vi "2 dof inverse.vi"() -> ()   [LabVIEW 2021]
panel:
  out "Motor angles":cluster{"x":dbl, "y":dbl, "x 2":dbl, "y 2":dbl}
  in  "Parameters of 2 DOF":T1={"X"=0.0, "Y"=0.0, "l1"=230.59, "l2"=112.96, "phi (rad)"=112.96} caption="Parameters of Delta Robot"
  # "Definitions about the Inputs of Forward Kinematics :"
  # "Theta Motor 1 , Theta Motor 2 represents the angles of two smart motors of 2 DOF."
  # "l1 and l2 respresents links length."
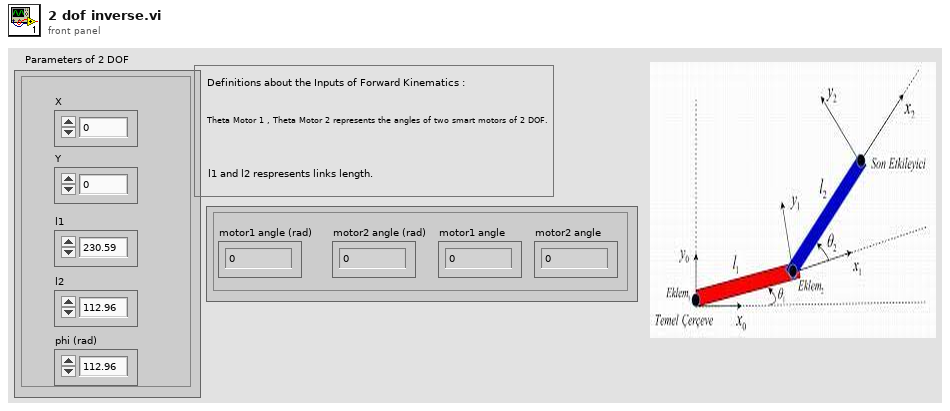
[diagram p1: front panel]
types:
  T1 = cluster{"X":dbl, "Y":dbl, "l1":dbl, "l2":dbl, "phi (rad)":dbl}
  T2 = cluster{"theta1":dbl, "theta2":dbl, "theta1_dg":dbl, "theta2_dg":dbl}
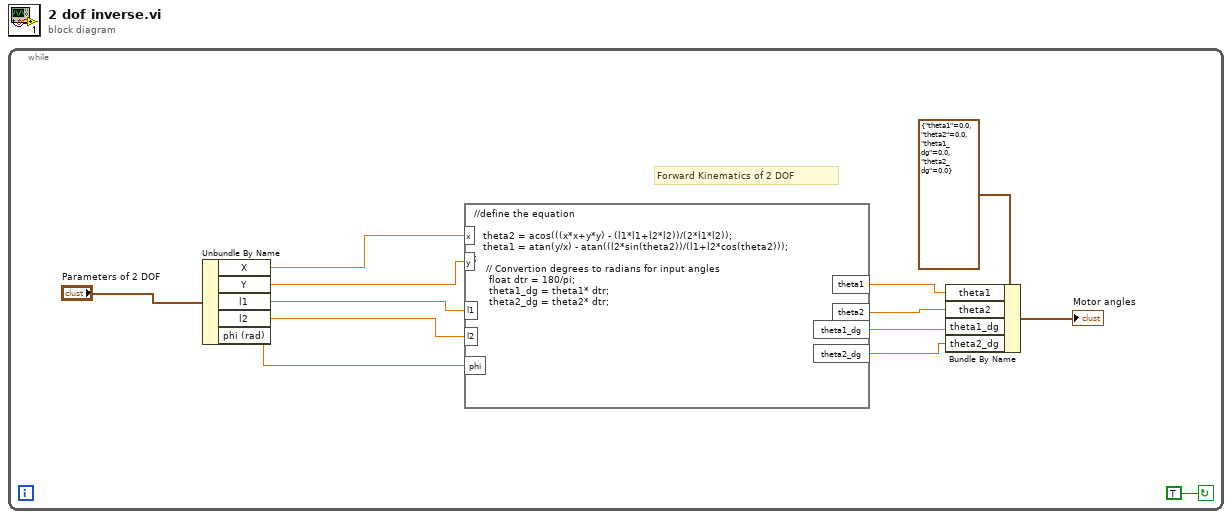
[diagram p0: block diagram]
diagram:
  n1 = while {
    stop <- TRUE continue-if-true
    # "Forward Kinematics of 2 DOF"
    n2 = Unbundle By Name "Unbundle By Name"("Parameters of 2 DOF") -> ("X"=w9:dbl, "Y"=w11:dbl, "l1"=w13:dbl, "l2"=w12:dbl, "phi (rad)"=w4:dbl)
    n3 = formula code="//define the equation\n\n   theta2 = acos(((x*x+y*y) - (l1*l1+l2*l2))/(2*l1*l2)); \n   theta1 = atan(y/x) - atan((l2*sin(theta2))/(l1+l2*cos(theta2)));\n;\n    // Convertion degrees to radians for input angles\n     float dtr = 180/pi;\n     theta1_dg = theta1* dtr;\n     theta2_dg = theta2* dtr;"("x"=w9, "y"=w11, "l1"=w13, "l2"=w12, "phi"=w4) -> ("theta1"=w8:dbl, "theta2"=w6:dbl, "theta1_dg"=w3:dbl, "theta2_dg"=w2:dbl)
    n4 = Bundle By Name(cluster=T2 {"theta1"=0.0, "theta2"=0.0, "theta1_dg"=0.0, "theta2_dg"=0.0}, "theta1"=w8, "theta2"=w6, "theta1_dg"=w3, "theta2_dg"=w2) -> (→"Motor angles":T2)
  }
